vi "3.vi"() -> ()   [LabVIEW 2013]
uses:
  <vilib>/Math Plots/3D Math Plots/3D Surface/3D Surface XCtrl/3D Surface.xctl
  <vilib>/Math Plots/3D Math Plots/3D Surface/3D Surface Datatype/Public/Plot Helper (Matrix).vi
  <vilib>/express/express arith-compare/Formula/XNode/ExpressFormulaBlockNode.xnode
  <vilib>/Math Plots/3D Math Plots/3D Surface/3D Surface Datatype/3D Surface Datatype.lvclass
panel:
  out "3D Surface":refnum<class "3D Plot Datatype.lvclass">[](xcontrol)
  in  "r":dbl
  in  "R":dbl
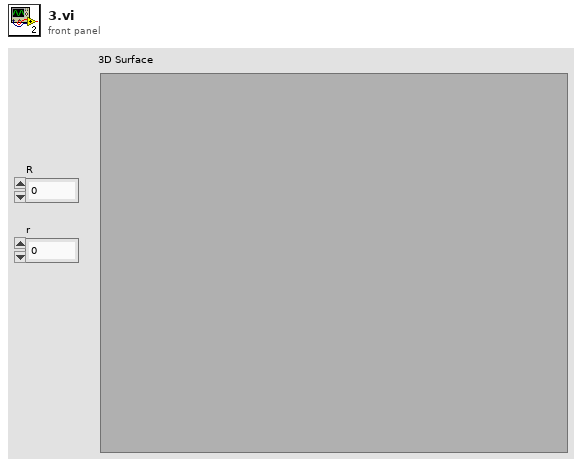
[diagram p1: front panel]
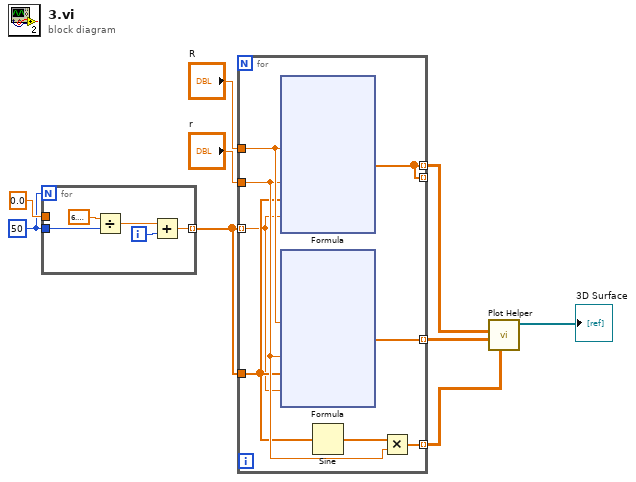
[diagram p0: block diagram]
diagram:
  w8 = 50
  n1 = for {
    N: w8 -> [_]
    tunnel: 0.0 -> [_]
    tunnel: w8 -> [w13]
    tunnel: [w10] -> w4 mode=indexing
    i -> [w11]
    n2 = Divide(x=6.283185307179586, y=w13) -> (x/y=w12:dbl)
    n3 = Add(x=w12, y=w11) -> (x+y=w10:dbl)
  }
  n4 = for {
    tunnel: "R" -> [w19]
    tunnel: w4 -> [w17]
    tunnel: "r" -> [w18]
    tunnel: [w20] -> _ mode=indexing
    tunnel: w4 -> [w16] mode=indexing
    tunnel: [w21] -> w3 mode=indexing
    tunnel: [w20] -> w2 mode=indexing
    tunnel: [w15] -> w1 mode=indexing
    n5 = xnode "Formula"("R"=w19, "r"=w18, "alfa"=w17, "beta"=w16) -> ("Result"=w20:dbl[])  [unwired: 1 in, 1 out]
    n6 = xnode "Formula"("R"=w19, "r"=w18, "alfa"=w17, "beta"=w16) -> ("Result"=w15:dbl[])  [unwired: 1 in, 1 out]
    n7 = Sine(x=w17) -> (sin(x)=w22:dbl[])
    n8 = Multiply(x=w22, y=w18) -> (x*y=w21:dbl[])
  }
  n9 = call-poly <vilib>:"Plot Helper.vi"("z matrix"=w3, "y matrix"=w1, "x matrix"=w2) -> ("3D Plot lvclass Array out"=→"3D Surface":refnum<class "3D Plot Datatype.lvclass">[])  [unwired: 3 in, 5 out]
